vi "Create Log File Path.vi"(8 "error in (no error)":errorcluster, 11 "File Storage Settings":T1={"Data Repository"=path "M:/data", "File Name Prefix (no spaces)"="logger", "Approximate File Size (kB)"=1000.0}) -> (0 "error out":errorcluster, 3 "Path":path)   [LabVIEW 2018, in "S3DK.lvlib"]
doc: "Statnett PMU Reference Library\nCreates a Log File Path depending on File Storage Settings"
uses:
  <vilib>/S3DK.lvlib
panel:
  # "INPUT"
  # "INTERMEDIATE"
  # "OUTPUT"
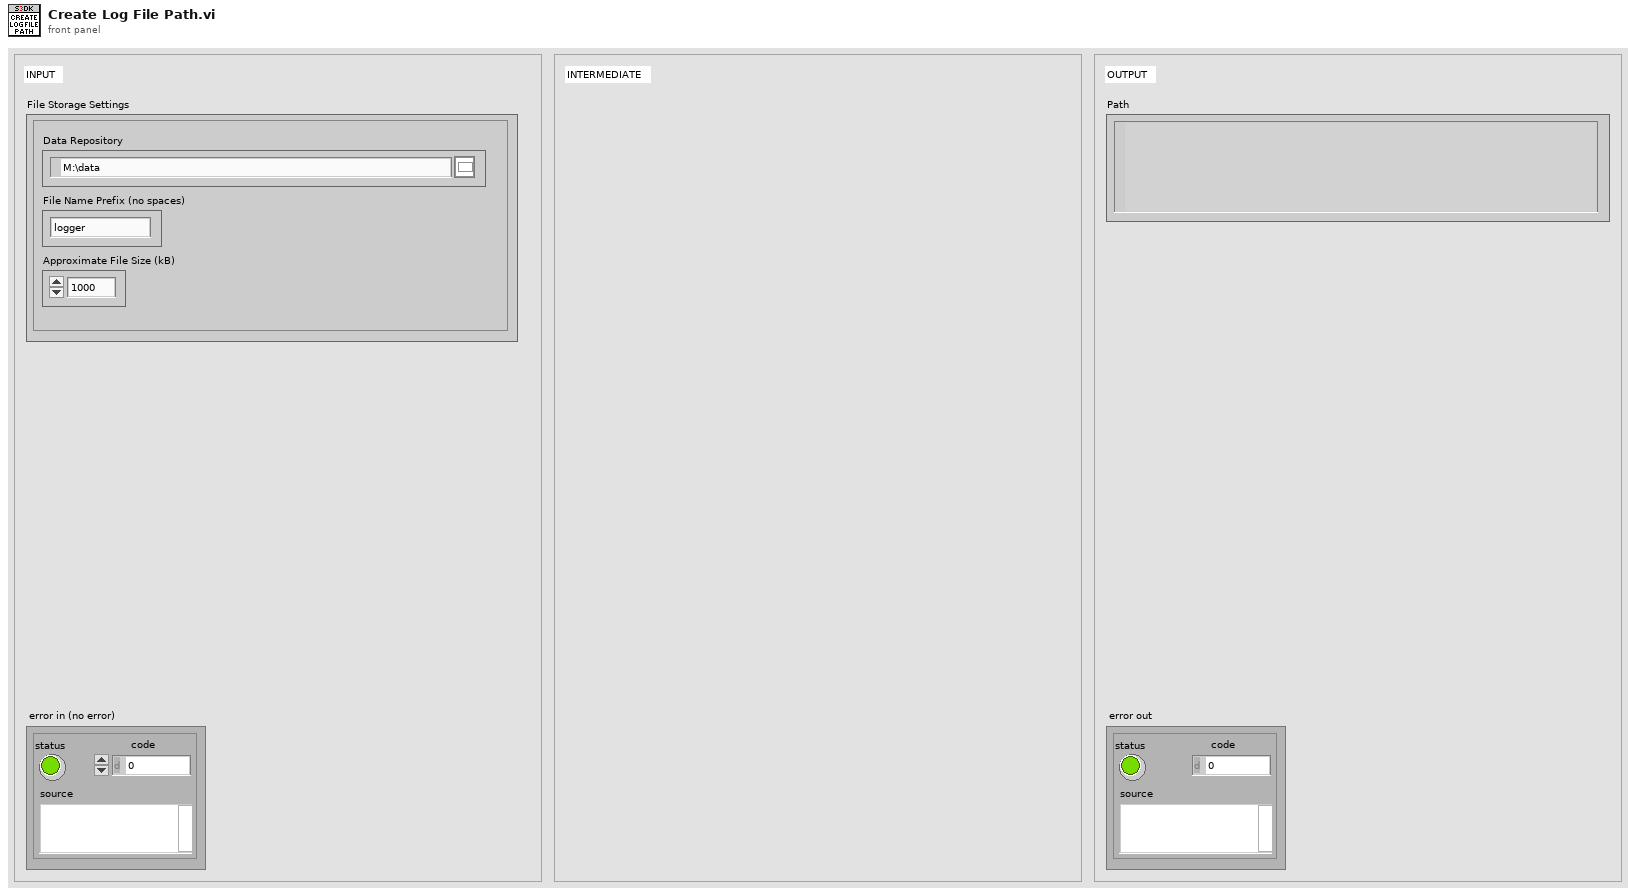
[diagram p1: front panel]
types:
  T1 = cluster{"Data Repository":path, "File Name Prefix (no spaces)":string, "Approximate File Size (kB)":dbl}
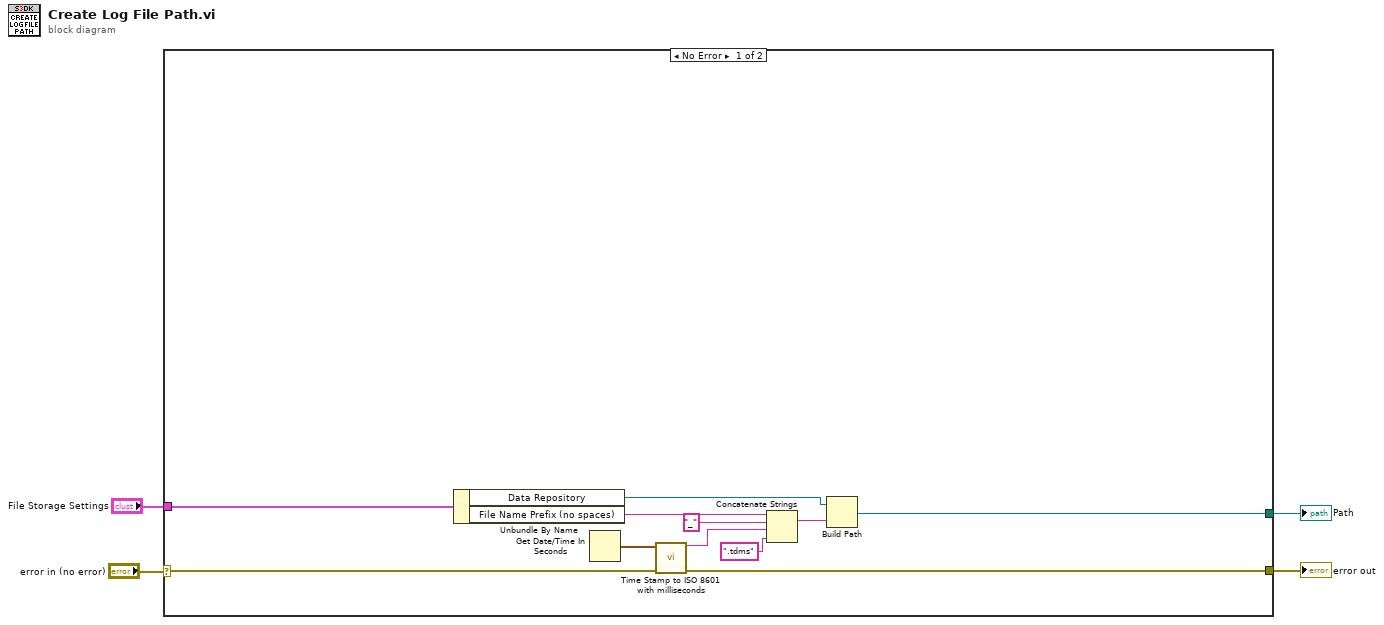
[diagram p0: block diagram]
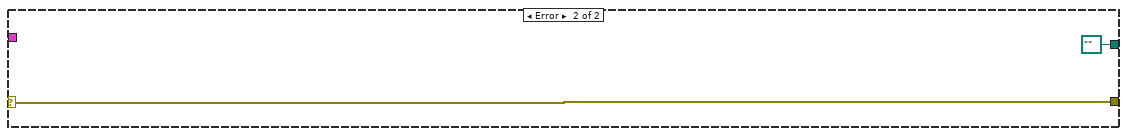
[diagram p2: hidden frame]
diagram:
  n1 = case shown="No Error" "error in (no error)" {
    selector: "error in (no error)" -> [w7 w17]
    tunnel: [w6 w17] -> w3
    tunnel: "File Storage Settings" -> [w8 _]
    tunnel: [w5 path "" ("appended path")] -> w1
    frame No Error {
      n2 = Unbundle By Name(w8) -> ("Data Repository"=w10:path, "File Name Prefix (no spaces)"=w12:string)
      n3 = Get Date/Time In Seconds() -> (seconds since 1Jan1904=w15:timestamp)
      n4 = call "Time Stamp to ISO 8601 with milliseconds.vi"("error in (no error)"=w7, "Timestamp"=w15) -> ("error out"=w6:errorcluster, "ISO 8601 w/ms"=w14:string)  [unwired: 8 in]
      n5 = Concatenate Strings(w12, "_" ("string"), w14, ".tdms" ("string")) -> (w11:string)
      n6 = Build Path(base path=w10, name or relative path=w11) -> (appended path=w5:path)
    }
    frame Error {
    }
  }
  "error out" <- w3
  "Path" <- w1
